vi "Set Device as Islanding Control.vi"(8 "error in (no error)":errorcluster, 11 "IED in":refnum<class "IED.lvclass">) -> (0 "error out":errorcluster, 3 "IED out":refnum<class "IED.lvclass">)   [LabVIEW 2015, in "IED Actor.lvlib" / "IED.lvclass"]
uses:
  IED.lvclass
  <vilib>/ActorFramework/Actor/Actor.lvclass/Actor.ctl
  IED.lvclass/IED.ctl
  SCADA Core/SCADA Abstract Messages/Device Action Status Msg/Device Action Status.ctl
  SCADA Core/SCADA Response Messages/Return Island Control Status Msg/Return Island Control Status Msg.lvclass/Return Island Control Status Msg.ctl
  <vilib>/ActorFramework/Message Enqueuer/Message Enqueuer.lvclass/Message Enqueuer.ctl
  <vilib>/NI/Tools/Keyed Array/Map String.vi
  <vilib>/ActorFramework/Message Enqueuer/Enqueue.vi
  <vilib>/NI/Tools/String/Get Case Matching.vi
  <vilib>/ActorFramework/Message Priority Queue/Priority Enqueue.vi
  SCADA Core/SCADA Response Messages/Return Island Control Status Msg/Return Island Control Status Msg.lvclass
  <vilib>/Modbus/master/Modbus Master.lvclass
  <vilib>/NI/Tools/Keyed Array/Tools_KeyedArray.lvlib
  <vilib>/ActorFramework/Actor/Actor.lvclass
  Utilities/Message Strings.llb/Message String Utilities.lvlib
  SCADA Core/SCADA Abstract Messages/Device Action Status Msg/Device Action Status Msg.lvclass
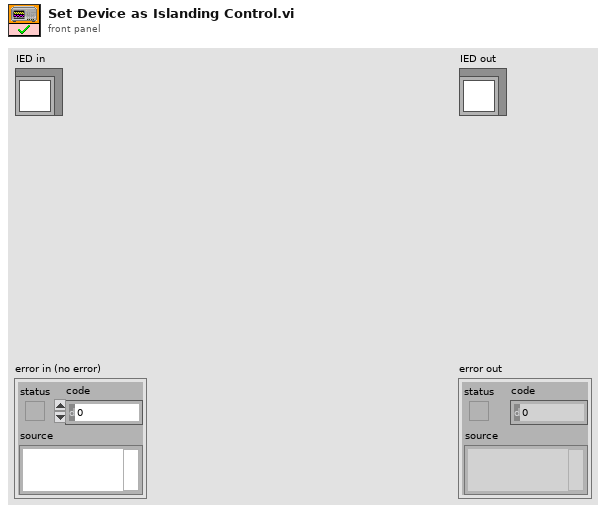
[diagram p1: front panel]
types:
  T1 = typedef "SCADA Core.lvlib/Device Action Status Msg.lvclass/Device Action Status.ctl" = enum16{"Success", "Failure"}
  T2 = typedef "Tools_KeyedArray.lvlib/KeyedArray.ctl" = cluster{"keys":string[], "values":string[]}
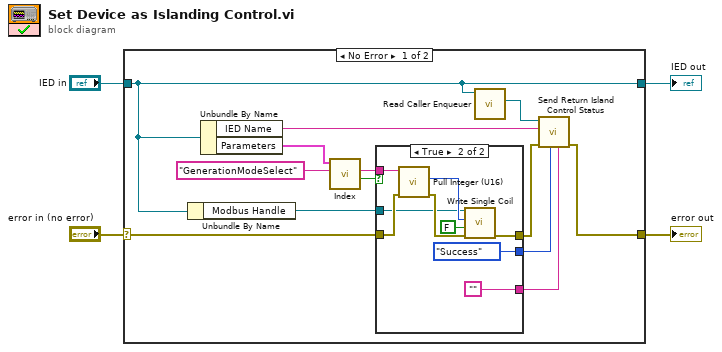
[diagram p0: block diagram]
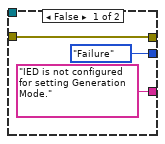
[diagram p2: hidden frame]
diagram:
  n1 = case shown="No Error" "error in (no error)" {
    selector: "error in (no error)" -> [w6 w31]
    tunnel: [w5 w31] -> w3
    tunnel: [w8 w30] -> w1
    tunnel: "IED in" -> [w8 w30]
    frame No Error {
      n2 = Unbundle By Name(w8) -> ("Modbus Handle"=w7:refnum<class "Modbus Master.lvclass">)
      n3 = Unbundle By Name(w8) -> ("IED Name"=w12:string, "Parameters"=w17:T2)
      n4 = call <vilib>:"Index.vi"("key"="GenerationModeSelect", "array in"=w17) -> ("valid key"=w15:bool, "value"=w13:string)  [unwired: 3 in, 1 out]
      n5 = case shown="True" w15 {
        tunnel: w13 -> [_ w29]
        tunnel: w6 -> [w20 w28]
        tunnel: [w20 w24] -> w11
        tunnel: [Device_Action_Status."Failure" ("Status") Device_Action_Status."Success" ("Status")] -> w10
        tunnel: ["IED is not configured for setting Generation Mode." ("error string") "" ("error string")] -> w9
        tunnel: w7 -> [_ w21]
        frame False {
        }
        frame True {
          n6 = call "Pull Integer (U16).vi"("error in (no error)"=w28, "String in"=w29) -> ("error out"=w27:errorcluster, "Integer out"=w26:u16)  [unwired: 7 in, 1 out]
          n7 = call-dynamic "Write Single Coil.vi"("error in (no error)"=w27, "coil value"=FALSE, "address"=w26, "Modbus master in"=w21) -> ("error out"=w24:errorcluster)  [unwired: 6 in, 1 out]
        }
      }
      n8 = call <vilib>:"Read Caller Enqueuer.vi"("Actor"=w8) -> ("Caller Enqueuer"=w14:refnum<class "Message Enqueuer.lvclass">)  [unwired: 10 in]
      n9 = call "Send Return Island Control Status.vi"("error string"=w9, "Status"=w10, "error in (no error)"=w11, "IED Name"=w12, "Message Enqueuer"=w14) -> ("error out"=w5:errorcluster)  [unwired: 5 in, 1 out]
    }
    frame Error {
    }
  }
  "error out" <- w3
  "IED out" <- w1
